vi "Set and Get Disp .vi"(7 "Mode":T1, 8 "错误输入":errorcluster, 10 "显示项输入":T3, 11 "Listbox Ref":refnum<vi>) -> (0 "错误输出":errorcluster, 2 "显示项输出":T2, 3 "Dup Listbox Ref":refnum<vi>)   [LabVIEW 2011, in "Listbox Tool.lvlib"]
uses:
  Listbox Tool.lvlib
  Custom Type/Disp.ctl
  Custom Type/Read and Write Mode.ctl
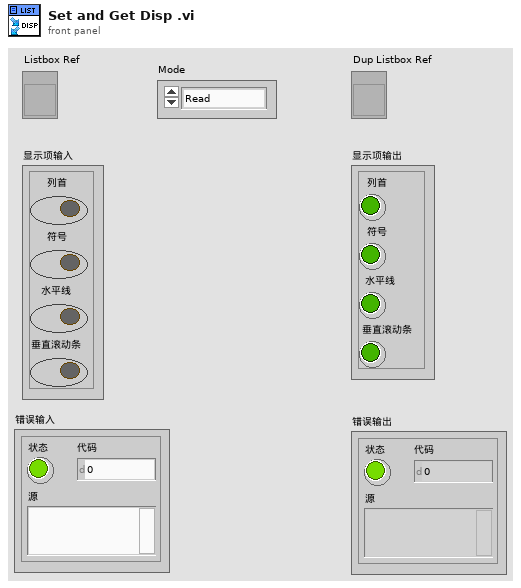
[diagram p1: front panel]
types:
  T1 = typedef "Listbox Tool.lvlib/Read and Write Mode.ctl" = enum16{"Read", "Write"}
  T2 = cluster{"列首":bool, "符号":bool, "水平线":bool, "垂直滚动条":bool}
  T3 = typedef "Listbox Tool.lvlib/Disp.ctl" = cluster{"列首":bool, "符号":bool, "水平线":bool, "垂直滚动条":bool}
  T4 = cluster{"ColHdrVis":bool, "Symbols Visible":bool, "Horizontal Lines Visible":bool, "Scrollbar Visible":bool}
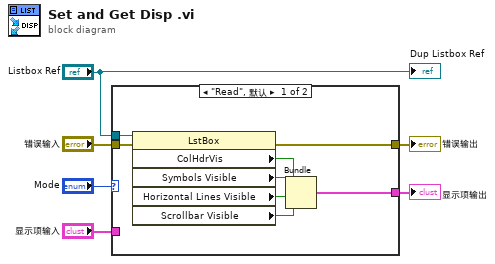
[diagram p0: block diagram]
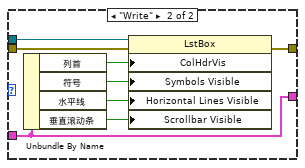
[diagram p2: hidden frame]
diagram:
  n1 = case shown="\"Read\", 默认" "Mode" {
    tunnel: [w10 w19] -> w5
    tunnel: "显示项输入" -> [_ w19]
    tunnel: "错误输入" -> [w9 w22]
    tunnel: [w8 w20] -> w2
    tunnel: "Listbox Ref" -> [w7 w21]
    frame "Read", Default {
      n2 = property class="LstBox"(reference=w7, error in=w9) -> (error out=w8:errorcluster, "ColHdrVis"=w14:bool, "Symbols Visible"=w13:bool, "Horizontal Lines Visible"=w12:bool, "Scrollbar Visible"=w11:bool)  [unwired: 1 out]
      n3 = Bundle("ColHdrVis"=w14, "Symbols Visible"=w13, "Horizontal Lines Visible"=w12, "Scrollbar Visible"=w11) -> (w10:T4)  [unwired: 1 in]
    }
    frame "Write" {
      n4 = Unbundle By Name(w19) -> ("列首"=w18:bool, "符号"=w17:bool, "水平线"=w16:bool, "垂直滚动条"=w15:bool)
      n5 = property class="LstBox"(reference=w21, error in=w22, "ColHdrVis"=w18, "Symbols Visible"=w17, "Horizontal Lines Visible"=w16, "Scrollbar Visible"=w15) -> (error out=w20:errorcluster)  [unwired: 1 out]
    }
  }
  "显示项输出" <- w5
  "错误输出" <- w2
  "Dup Listbox Ref" <- "Listbox Ref"
